vi "test_generate_midi_event.vi"(8 "error in (no error)":errorcluster, 10 "user event out":refnum<user-event>, 11 "LabVIEW-MIDI-XPLAT in":refnum<class "LabVIEW-MIDI-XPLAT.lvclass">) -> (0 "error out":errorcluster, 2 "Return":i32, 3 "LabVIEW-MIDI-XPLAT out":refnum<class "LabVIEW-MIDI-XPLAT.lvclass">)   [LabVIEW 2020, in "LabVIEW-MIDI-XPLAT.lvclass"]
uses:
  LabVIEW-MIDI-XPLAT.lvclass
  LabVIEW-MIDI-XPLAT.lvclass/LabVIEW-MIDI-XPLAT.ctl
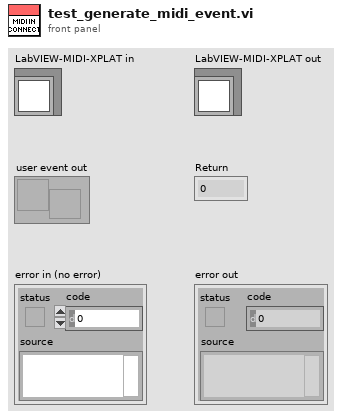
[diagram p1: front panel]
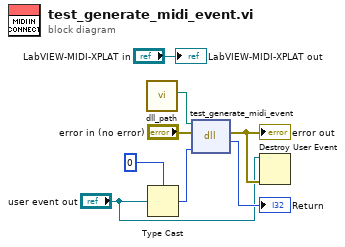
[diagram p0: block diagram]
diagram:
  n1 = call "dll_path.vi"() -> ("dll"=w5:path)  [unwired: 11 in]
  n2 = Type Cast(type=u32 0, x="user event out") -> (*(type *) &x=w3:u32)
  n3 = dll-call lib="C:/code/LabVIEW-MIDI-XPLAT/dist/TomMIDIllan_*.*" fn="test_generate_midi_event"(path in=w5, error in="error in (no error)", "user_event_ref"=w3) -> (error out=w2:errorcluster, "handle"=→"Return":i32)  [unwired: 2 in, 1 out]
  "error out" <- w2
  n4 = Destroy User Event(user event="user event out", error in=w2) -> ()  [unwired: 1 out]
  "LabVIEW-MIDI-XPLAT out" <- "LabVIEW-MIDI-XPLAT in"
